vi "_Remote Communicate.vi"(4 "String":string, 5 "Max Mass":dbl, 6 "error in (no error)":errorcluster, 7 "DC Param":u16, 8 "Parameter":T1 {"Expt"."Mass Range"."Resolution Type" items=["High/High", "Medium/Medium", "Low/Low", "High/Medium", "High/Low", "Medium/High", "Medium/Low", "Low/High", "Low/Medium"]}, 9 "Command":T7=enum."Get Info") -> (0 "error out":errorcluster, 1 "Data Array":i32[](array[numeric]), 2 "Info":string, 3 "CommErr":bool)   [LabVIEW 2015]
uses:
  Type/_RT Data.ctl
  Type/_RT Command.ctl
  Type/_RT Parameter.ctl
  Type/_RT Active Ch.ctl
  Type/_RT Expt.ctl
  Type/_Run Mode.ctl
  Type/_RT Mass Range.ctl
  Type/_RT Res Type.ctl
  Type/TCP Packet Info.ctl
  Type/_File Command.ctl
  Type/_RT Configuration 2.ctl
  Type/_Log Command.ctl
  Configuration/_Global Configuration.vi
  <vilib>/Utility/config.llb/Read Key (String).vi
  <vilib>/Utility/config.llb/NI_LVConfig.lvlib
panel:
  out "Boolean":bool
  in  "Data":T8
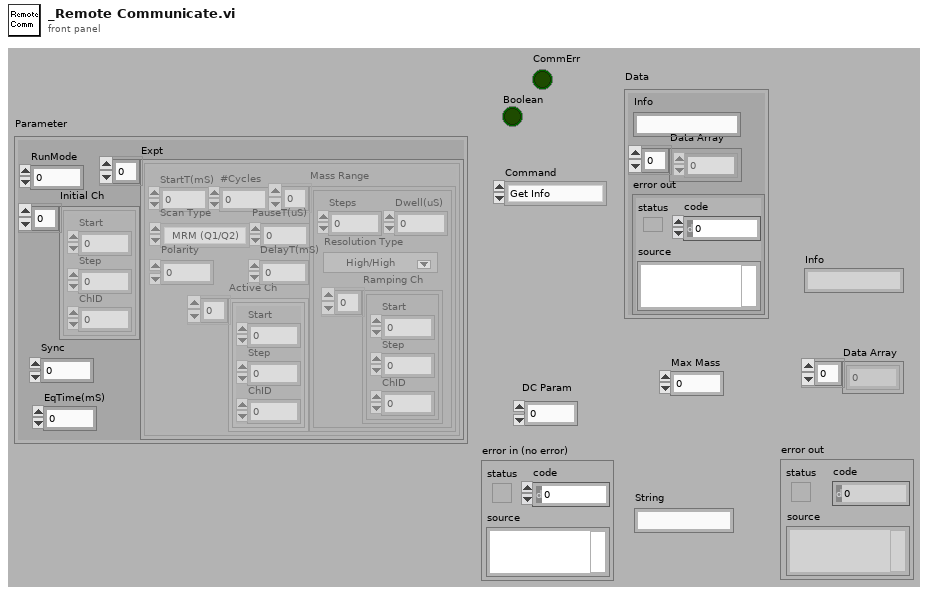
[diagram p1: front panel]
types:
  T1 = typedef "_RT Parameter.ctl" = cluster{"RunMode":i32, "Initial Ch":T2[], "Sync":u8, "Expt":T3[], "EqTime(mS)":i32}
  T2 = typedef "_RT Active Ch.ctl" = cluster{"Start":i32, "Step":i32, "ChID":i32}
  T3 = typedef "_RT Expt.ctl" = cluster{"StartT(mS)":i32, "#Cycles":i32, "Scan Type":T4, "PauseT(uS)":i32, "Polarity":u8, "DelayT(mS)":i32, "Active Ch":T2[], "Mass Range":T5[]}
  T4 = typedef "_Run Mode.ctl" = enum16{"MRM (Q1/Q2)", "Q1 Scan", "Q1 SRM", "Q2 Scan", "Q2 SRM", "Product Scan", "Precursor Scan", "Neutral Loss", "Neutral Gain"}
  T5 = typedef "_RT Mass Range.ctl" = cluster{"Steps":i32, "Dwell(uS)":i32, "Resolution Type":T6, "Ramping Ch":T2[]}
  T6 = typedef "_RT Res Type.ctl" = u16
  T7 = typedef "_RT Command.ctl" = enum16{"xml Start Run", "xml Start Actual Run", "xml Stop Run", "xml Runtime Update", "xml Get Status", "xml Get Table", "xml Set Table", "xml Get Configuration", "xml System Status", "xml Set LC Input Logic", "xml Get Data", "xml Get Info", "Start", "StartActualRun", "Stop", "Runtime Update", "Get Data", "Get Info", "Get Status", "Get Param", "Get Config", "Get Table", "Read ADC", "Set Oscillator", "Update Config", "Update Table", "Set All Pol", "Set Pol and DC", "Set Max Mass", "Toggle RP", "Toggle EL", "Set PIC", "Initialize Turbo", "Send Turbo Comm", "Close Turbo", "P1", "P2", "P3", "Send Serial", "Set LC Out", "Get LC In", "Read VAC", "Test Table", "Toggle Power", "Get Startup", "Set Startup", "Get ADC Table", "Set ADC Table", "Get Brief Status", "Get Detail Status", "Auxiliary Update", "Set CC Logics", "Set CC Input Logics", "Ignore Error", "invalid"}
  T8 = typedef "_RT Data.ctl" = cluster{"Info":string, "Data Array":i32[], "error out":errorcluster}
  T9 = typedef "TCP Packet Info.ctl" = cluster{"Packet Signature":string, "Sequence Number":i32, "Command":T7, "Data Message Size":u32, "Data Message Size":string, "Data Message":string, "Error Message Size":u32, "Error Message Size":string, "Error Message":string, "Checksum":u32, "Error Message":errorcluster, "Command ID":string}
  T10 = typedef "_File Command.ctl" = enum16{"No Command", "Open", "Open Read", "Write", "Get Spectrum", "Close"}
  T11 = typedef "_RT Configuration 2.ctl" = cluster{"Name":string, "Ch#":u8, "Min":dbl, "Max":dbl, "Def+":dbl, "Def-":dbl, "Offset":dbl, "Slope":dbl, "Type":u8, "Description":string, "SettleT":dbl}
  T12 = typedef "_RT Instrument 2.ctl" = cluster{"Table":T11[], "Instrument":string[]}
  T13 = typedef "NI_LVConfig.lvlib/Config Data RefNum.ctl" = refnum<k1>
  T14 = typedef "_Log Command.ctl" = enum16{"No Command", "Open", "Read", "Write", "Close", "Check Size"}
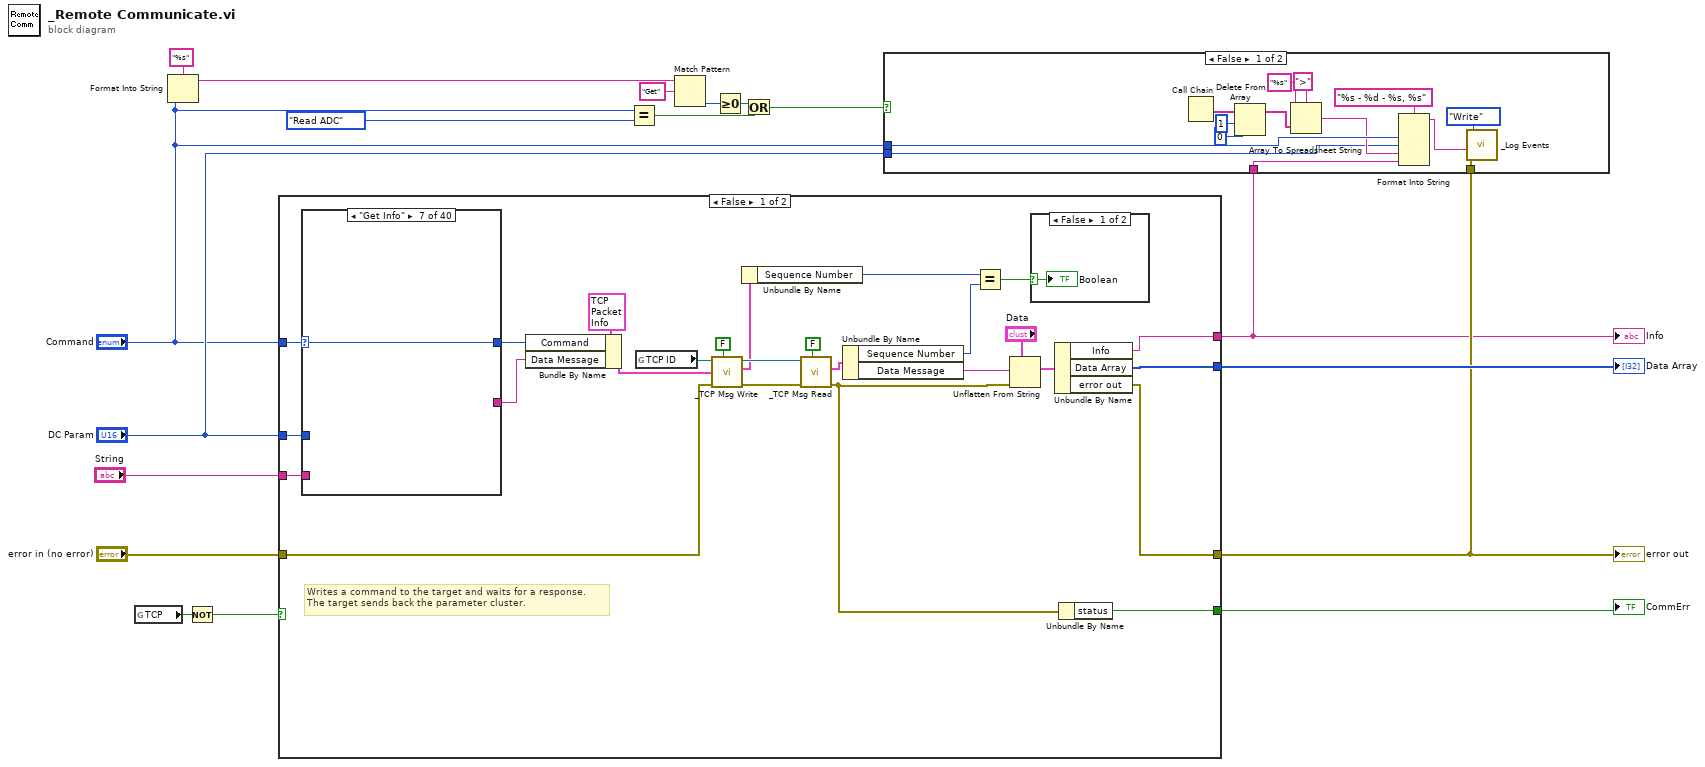
[diagram p0: block diagram]
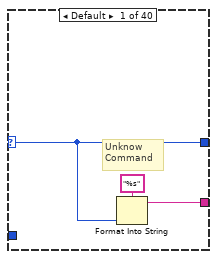
[diagram p4: hidden frame]
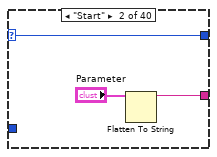
[diagram p5: hidden frame]
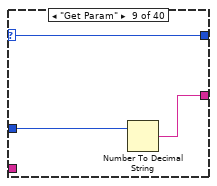
[diagram p11: hidden frame]
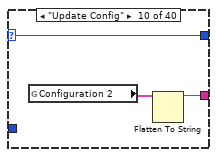
[diagram p12: hidden frame]
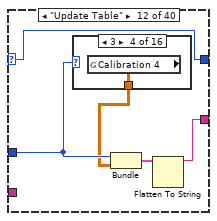
[diagram p14: hidden frame]
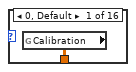
[diagram p15: hidden frame]
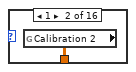
[diagram p16: hidden frame]
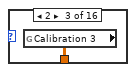
[diagram p17: hidden frame]
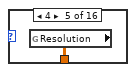
[diagram p18: hidden frame]
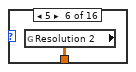
[diagram p19: hidden frame]
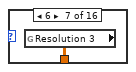
[diagram p20: hidden frame]
diagram:
  n1 = global read "_Global Configuration.vi" "TCP"() -> (w18:bool)
  n2 = Format Into String(format string="%s", "Command") -> (resulting string=w10:string)  [unwired: 2 in, 1 out]
  n3 = Not(x=w18) -> (.not. x?=w15:bool)
  n4 = case shown="False" w15 {
    selector: w15 -> [_ w151]
    tunnel: [w37 w156] -> w14
    tunnel: "error in (no error)" -> [w33 w156]
    tunnel: [w40 w154] -> w12
    tunnel: [w39 w153] -> w16
    tunnel: "Command" -> [w31 w155]
    tunnel: "DC Param" -> [w38 w152]
    tunnel: [w36 w151] -> w2
    tunnel: "String" -> [w35 _]
    frame False {
      # "Writes a command to the target and waits for a response.\nThe target sends back the parameter cluster."
      n5 = case shown="\"Get Info\"" w31 {
        selector: w31 -> [w46 w49 w52 w53 w54 w56 w57 w58 w59 w62 w65 w66 w87 w90 w92 w93 w94 w96 w98 w99 w102 w105 w108 w111 w114 w115 w118 w121 w124 w126 w128 w131 w134 w137 w138 w140 w141 w143 w145 w148]
        tunnel: [w47 w51 _ _ w55 _ _ _ w60 w63 _ w70 w88 w91 _ _ w95 w97 _ w100 w103 w107 w110 w113 _ w116 w119 w122 w125 w127 w130 w133 w136 _ w139 _ w142 w144 w147 w149] -> w29
        tunnel: w38 -> [_ _ _ _ _ _ _ _ w61 _ _ w68 w89 _ _ _ _ _ _ w101 w104 w106 w109 w112 _ w117 w120 w123 _ _ w129 w132 w135 _ _ _ _ _ _ w150]
        tunnel: w35 -> [_ _ _ _ w55 _ _ _ _ _ _ _ _ w91 _ _ w95 w97 _ _ _ _ _ _ _ _ _ _ w125 w127 _ _ _ _ w139 _ w142 w144 _ _]
        tunnel: [w46 w49 w52 w53 w54 w56 w57 w58 w59 w62 w65 w66 w87 w90 w92 w93 w94 w96 w98 w99 w102 w105 w108 w111 w114 w115 w118 w121 w124 w126 w128 w131 w134 w137 w138 w140 w141 w143 w145 w148] -> w28
        frame Default {
          # "Unknow\nCommand"
          n6 = Format Into String(format string="%s", w46) -> (resulting string=w47:string)  [unwired: 2 in, 1 out]
        }
        frame "Start" {
          n7 = Flatten To String(anything="Parameter") -> (data string=w51:string)  [unwired: 1 in, 4 out]
        }
        frame "StartActualRun" {
        }
        frame "Stop" {
        }
        frame "Runtime Update" {
        }
        frame "Get Data" {
        }
        frame "Get Info" {
        }
        frame "Get Status" {
        }
        frame "Get Param" {
          n8 = Number To Decimal String(number=w61) -> (decimal integer string=w60:string)  [unwired: 1 out]
        }
        frame "Update Config" {
          n9 = global read "_Global Configuration.vi" "Configuration 2"() -> (w64:T12)
          n10 = Flatten To String(anything=w64) -> (data string=w63:string)  [unwired: 1 in, 4 out]
        }
        frame "Get Config" {
        }
        frame "Update Table" {
          n11 = case shown="3" w68 {
            tunnel: [w71 w72 w73 w74 w75 w76 w77 w78 w79 w80 w81 w82 w83 w84 w85 w86] -> w67
            frame 0, Default {
              n12 = global read "_Global Configuration.vi" "Calibration"() -> (w71:dbl[][])
            }
            frame 1 {
              n13 = global read "_Global Configuration.vi" "Calibration 2"() -> (w72:dbl[][])
            }
            frame 2 {
              n14 = global read "_Global Configuration.vi" "Calibration 3"() -> (w73:dbl[][])
            }
            frame 3 {
              n15 = global read "_Global Configuration.vi" "Calibration 4"() -> (w74:dbl[][])
            }
            frame 4 {
              n16 = global read "_Global Configuration.vi" "Resolution"() -> (w75:dbl[][])
            }
            frame 5 {
              n17 = global read "_Global Configuration.vi" "Resolution 2"() -> (w76:dbl[][])
            }
            frame 6 {
              n18 = global read "_Global Configuration.vi" "Resolution 3"() -> (w77:dbl[][])
            }
            frame 7 {
              n19 = global read "_Global Configuration.vi" "Resolution 4"() -> (w78:dbl[][])
            }
            frame 8 {
              n20 = global read "_Global Configuration.vi" "Resolution 5"() -> (w79:dbl[][])
            }
            frame 9 {
              n21 = global read "_Global Configuration.vi" "Resolution 6"() -> (w80:dbl[][])
            }
            frame 10 {
              n22 = global read "_Global Configuration.vi" "Resolution 7"() -> (w81:dbl[][])
            }
            frame 11 {
              n23 = global read "_Global Configuration.vi" "Resolution 8"() -> (w82:dbl[][])
            }
            frame 12 {
              n24 = global read "_Global Configuration.vi" "Resolution 9"() -> (w83:dbl[][])
            }
            frame 13 {
              n25 = global read "_Global Configuration.vi" "Resolution 10"() -> (w84:dbl[][])
            }
            frame 14 {
              n26 = global read "_Global Configuration.vi" "Resolution 11"() -> (w85:dbl[][])
            }
            frame 15 {
              n27 = global read "_Global Configuration.vi" "Resolution 12"() -> (w86:dbl[][])
            }
          }
          n28 = Bundle("DC Param"=w68, "Resolution 12"=w67) -> (w69:cluster{"DC Param":u16, "Resolution 12":dbl[][]})  [unwired: 1 out]
          n29 = Flatten To String(anything=w69) -> (data string=w70:string)  [unwired: 1 in, 4 out]
        }
        frame "Get Table" {
          n30 = Number To Decimal String(number=w89) -> (decimal integer string=w88:string)  [unwired: 1 out]
        }
        frame "Set ADC Table" {
        }
        frame "Get ADC Table" {
        }
        frame "Read ADC" {
        }
        frame "Set Oscillator" {
        }
        frame "Set Startup" {
        }
        frame "Get Startup" {
        }
        frame "Set All Pol" {
          n31 = Type Cast(x=w101) -> (*(type *) &x=w100:string)  [unwired: 1 out]
        }
        frame "Set Pol and DC" {
          n32 = Type Cast(x=w104) -> (*(type *) &x=w103:string)  [unwired: 1 out]
        }
        frame "P1" {
          n33 = Type Cast(x=w106) -> (*(type *) &x=w107:string)  [unwired: 1 out]
        }
        frame "P2" {
          n34 = Type Cast(x=w109) -> (*(type *) &x=w110:string)  [unwired: 1 out]
        }
        frame "P3" {
          n35 = Type Cast(x=w112) -> (*(type *) &x=w113:string)  [unwired: 1 out]
        }
        frame "Read VAC" {
        }
        frame "Toggle Power" {
          n36 = Number To Decimal String(number=w117) -> (decimal integer string=w116:string)  [unwired: 1 out]
        }
        frame "Toggle RP" {
          n37 = Number To Decimal String(number=w120) -> (decimal integer string=w119:string)  [unwired: 1 out]
        }
        frame "Toggle EL" {
          n38 = Number To Decimal String(number=w123) -> (decimal integer string=w122:string)  [unwired: 1 out]
        }
        frame "Set PIC" {
        }
        frame "Send Serial" {
        }
        frame "Set LC Out" {
          n39 = Type Cast(x=w129) -> (*(type *) &x=w130:string)  [unwired: 1 out]
        }
        frame "Set CC Logics" {
          n40 = Type Cast(x=w132) -> (*(type *) &x=w133:string)  [unwired: 1 out]
        }
        frame "Set CC Input Logics" {
          n41 = Type Cast(x=w135) -> (*(type *) &x=w136:string)  [unwired: 1 out]
        }
        frame "Get LC In" {
        }
        frame "Get Brief Status" {
        }
        frame "Get Detail Status" {
        }
        frame "Auxiliary Update" {
        }
        frame "Test Table" {
        }
        frame "Set Max Mass" {
          n42 = Type Cast(x="Max Mass") -> (*(type *) &x=w147:string)  [unwired: 1 out]
        }
        frame "Ignore Error" {
          n43 = Number To Decimal String(number=w150) -> (decimal integer string=w149:string)  [unwired: 1 out]
        }
      }
      n44 = Bundle By Name(cluster=T9 {"Packet Signature"="", "Sequence Number"=0, "Command"=enum."xml Set LC Input Logic", "Data Message Size"=0, "Data Message Size"="", "Data Message"="", "Error Message Size"=0, "Error Message Size"="", "Error Message"="", "Checksum"=0, "Error Message"={"status"=FALSE, "code"=0, "source"=""}, "Command ID"=""} ("Packet Info In"), "Command"=w28, "Data Message"=w29) -> (w27:T9)
      n45 = global read "_Global Configuration.vi" "TCP ID"() -> (w44:refnum<k5>)
      n46 = call "_TCP Msg Write.vi"("RT"=FALSE, "error in"=w33, "Packet Info In"=w27, "connection ID In"=w44) -> ("error out"=w21:errorcluster, "Packet Info In Out"=w22:T9, "connection ID out"=w42:refnum<k5>)  [unwired: 1 in, 4 out]
      n47 = Unbundle By Name(w22) -> ("Sequence Number"=w25:i32)
      n48 = call "_TCP Msg Read.vi"("RT"=FALSE, "error in"=w21, "connection ID"=w42) -> ("error out"=w19:errorcluster, "Packet Info"=w20:T9)  [unwired: 2 in, 5 out]
      n49 = Unbundle By Name(w20) -> ("Sequence Number"=w24:i32, "Data Message"=w34:string)
      n50 = Equal?(x=w25, y=w24) -> (x = y?=w23:bool)
      n51 = Unflatten From String(type="Data", binary string=w34, error in (no error)=w19) -> (value=w41:T8)  [unwired: 4 out]
      n52 = case shown="False" w23 {
        selector: w23 -> [w45 _]
        frame False {
          "Boolean" <- w45
        }
        frame True {
        }
      }
      n53 = Unbundle By Name(w41) -> ("Info"=w40:string, "Data Array"=w39:i32[], "error out"=w37:errorcluster)
      n54 = Unbundle By Name(w19) -> ("status"=w36:bool)
    }
    frame True {
      # "For simulation"
      n55 = case shown="\"Get Status\"" w155 {
        tunnel: [_ _ "Ionica is running in simulation mode.\n(System is idling: 00h00m00s)" w164 w172 "0\t118061205\tSimilated FPGA is idling\r\n4\t0\tFIFO Mis-Read #\r\n5\t4228\t# of Recorded Data Points\r\n6\t1451\tTime to Prepare Next Cycle (ticks)\r\n7\t14\tTotal # of Experiments Ran\r\n0\t1\tSingle Mode\r\n1\t10\t# of Active Channels\r\n2\t1000000\tHigh Level Time (uS)\r\n3\t500000\tLow Level Time (uS)" ("Info") w190 _ w199 w209] -> w154
        tunnel: [_ w157 _ _ _ _ _ w192 _ _] -> w153
        tunnel: w152 -> [_ _ _ _ w171 _ _ _ _ _]
        frame Default {
        }
        frame "Get Data" {
          n56 = call "_File Server Simulation.vi"("FileCommand"=_File_Command."Get Spectrum") -> ("DataArray"=w157:i32[])  [unwired: 1 in, 1 out]
        }
        frame "Get Info" {
        }
        frame "Get Status" {
          n57 = global read "_Global Configuration.vi" "Run"() -> (w168:bool)
          n58 = global read "_Global Configuration.vi" "Acquiring"() -> (w160:bool)
          n59 = Select(t="1: Simulated FPGA is running" ("regular expression"), s=w168, f="0: Simulated FPGA is in idle state" ("regular expression")) -> (s? t:f=w165:string)
          n60 = Select(t="Running" ("regular expression"), s=w160, f="Ready" ("regular expression")) -> (s? t:f=w161:string)
          n61 = Format Into String(format string="%s.  Instr State = %s.", w165, w161) -> (resulting string=w164:string)  [unwired: 2 in, 1 out]
        }
        frame "Get Table" {
          n62 = case shown="6" w171 {
            tunnel: [w173 w174 w175 w176 w177 w178 w179 w180 w181 w182 w183 w184 w185 w186 w187 w188] -> w170
            frame 0, Default {
              n63 = global read "_Global Configuration.vi" "Calibration"() -> (w173:dbl[][])
            }
            frame 1 {
              n64 = global read "_Global Configuration.vi" "Calibration 2"() -> (w174:dbl[][])
            }
            frame 2 {
              n65 = global read "_Global Configuration.vi" "Calibration 3"() -> (w175:dbl[][])
            }
            frame 3 {
              n66 = global read "_Global Configuration.vi" "Calibration 4"() -> (w176:dbl[][])
            }
            frame 4 {
              n67 = global read "_Global Configuration.vi" "Resolution"() -> (w177:dbl[][])
            }
            frame 5 {
              n68 = global read "_Global Configuration.vi" "Resolution 2"() -> (w178:dbl[][])
            }
            frame 6 {
              n69 = global read "_Global Configuration.vi" "Resolution 3"() -> (w179:dbl[][])
            }
            frame 7 {
              n70 = global read "_Global Configuration.vi" "Resolution 4"() -> (w180:dbl[][])
            }
            frame 8 {
              n71 = global read "_Global Configuration.vi" "Resolution 5"() -> (w181:dbl[][])
            }
            frame 9 {
              n72 = global read "_Global Configuration.vi" "Resolution 6"() -> (w182:dbl[][])
            }
            frame 10 {
              n73 = global read "_Global Configuration.vi" "Resolution 7"() -> (w183:dbl[][])
            }
            frame 11 {
              n74 = global read "_Global Configuration.vi" "Resolution 8"() -> (w184:dbl[][])
            }
            frame 12 {
              n75 = global read "_Global Configuration.vi" "Resolution 9"() -> (w185:dbl[][])
            }
            frame 13 {
              n76 = global read "_Global Configuration.vi" "Resolution 10"() -> (w186:dbl[][])
            }
            frame 14 {
              n77 = global read "_Global Configuration.vi" "Resolution 11"() -> (w187:dbl[][])
            }
            frame 15 {
              n78 = global read "_Global Configuration.vi" "Resolution 12"() -> (w188:dbl[][])
            }
          }
          n79 = Flatten To String(anything=w170) -> (data string=w172:string)  [unwired: 1 in, 4 out]
        }
        frame "Get Param" {
        }
        frame "Get Config" {
          n80 = global read "_Global Configuration.vi" "Configuration 2"() -> (w191:T12)
          n81 = Flatten To String(anything=w191) -> (data string=w190:string)  [unwired: 1 in, 4 out]
        }
        frame "Read ADC" {
          n82 = for {
            N: 128 -> [_]
            tunnel: [w194] -> w192 mode=indexing
            n83 = Random Number (0-1)() -> (number: 0 to 1=w197:dbl)
            n84 = Multiply(x=w197, y=4096.0) -> (x*y=w195:dbl)
            n85 = To Long Integer(number=w195) -> (32bit integer=w194:i32)
          }
        }
        frame "Get Detail Status" {
          n86 = global read "_Global Configuration.vi" "Single Source"() -> (w201:bool)
          n87 = Select(t="<Data>\n<SystemStatus>\nInstrument State=Simulation;\nServer State=0;\nLC1 IN=0;\nLC2 IN=0;\nLC1 Out1=1;\nLC1 Out2=0;\nLC2 Out1=1;\nLC2 Out2=0;\nSystem Error=;\nVacuum Gauge=1;\nVacuum Pressure=1164.34;\nVacuum Error=No Error;\nForeline Pressure=-29.22;\nForeline Error=No Error;\nSource 1=ESI;\nNeb Gas1=385.03;\nAux Gas1=313.04;\nCurtain Gas=109.38;\nCC Gas=439.94;\nOut of Gas=0;\nHSID Temp=198.00;\nSource1 Temp=251.00;\nVoltage Output=1;\nExhaust Pressure=3752.31;\nQ2RF HS1 Temp=36.38;\nQ1RF HS1 Temp=40.53;\nM1RF HS1 Temp=37.11;\nQ2RF HS2 Temp=37.35;\nQ1RF HS2 Temp=40.77;\nM1RF HS2 Temp=36.62;\nCorona Current=0.00;\nHTR PS Current=8.23;\nQ1 Tuning DC=-7.15;\nQ2 Tuning DC=-8.26;\nM1RF Tuning DC=-5.58;\nDoor Interlock=1;\n24V=24;\n28V=28;\n-28V=-28;\n60V=59;\n15V=15;\n-15V=-15;\nLens Board 2 +5V=5;\nLens Board 2 -5V=-5;\nLens Board 1 +5V=5;\nLens Board 1 -5V=-5;\nSource Exhaust Valve=1;\n</SystemStatus>\n<Log>\n97:33:2, Starting Up\n97:33:3, Electronics ON\n97:33:11, System Pumping Down\n97:34:28, Roughing Pump Standby\n97:34:28, Turbo Startup\n97:34:31, Turbo Ready\n97:34:34, System Ready\n</Log>\n</Data>", s=w201, f="<Data>\n<SystemStatus>\nInstrument State=Simulation;\nServer State=0;\nLC1 IN=0;\nLC2 IN=0;\nLC1 Out1=1;\nLC1 Out2=0;\nLC2 Out1=1;\nLC2 Out2=0;\nSystem Error=;\nVacuum Gauge=1;\nVacuum Pressure=1164.34;\nVacuum Error=No Error;\nForeline Pressure=-29.22;\nForeline Error=No Error;\nSource 1=ESI;\nSource 2=APCI;\nNeb Gas1=385.03;\nNeb Gas2=0.00;\nAux Gas1=313.04;\nAux Gas2=0.00;\nCurtain Gas=109.38;\nCC Gas=439.94;\nOut of Gas=0;\nHSID Temp=198.00;\nSource1 Temp=251.00;\nSource2 Temp=106.00;\nVoltage Output=1;\nExhaust Pressure=3752.31;\nQ2RF HS1 Temp=36.38;\nQ1RF HS1 Temp=40.53;\nM1RF HS1 Temp=37.11;\nQ2RF HS2 Temp=37.35;\nQ1RF HS2 Temp=40.77;\nM1RF HS2 Temp=36.62;\nCorona Current=0.00;\nHTR PS Current=8.23;\nQ1 Tuning DC=-7.15;\nQ2 Tuning DC=-8.26;\nM1RF Tuning DC=-5.58;\nDoor Interlock=1;\n24V=24;\n28V=28;\n-28V=-28;\n60V=59;\n15V=15;\n-15V=-15;\nLens Board 2 +5V=5;\nLens Board 2 -5V=-5;\nLens Board 1 +5V=5;\nLens Board 1 -5V=-5;\nSource Exhaust Valve=1;\n</SystemStatus>\n<Log>\n97:33:2, Starting Up\n97:33:3, Electronics ON\n97:33:11, System Pumping Down\n97:34:28, Roughing Pump Standby\n97:34:28, Turbo Startup\n97:34:31, Turbo Ready\n97:34:34, System Ready\n</Log>\n</Data>") -> (s? t:f=w199:string)
        }
        frame "Get ADC Table" {
          n88 = call "_Open Preference File.vi"() -> ("error"=w205:errorcluster, "refnum"=w204:T13)  [unwired: 3 in, 3 out]
          n89 = for {
            N: 128 -> [_]
            tunnel: w204 -> [w218]
            tunnel: w205 -> [w217]
            tunnel: "ADC" ("section") -> [w216]
            tunnel: [w214] -> w208
            tunnel: [w212] -> w202 mode=indexing
            i -> [w213]
            n90 = for {
              N: 8 -> [_]
              tunnel: w218 -> [w228]
              tunnel: w217 -> [w227]
              tunnel: w216 -> [w220]
              tunnel: [w226] -> w214
              tunnel: w213 -> [w224]
              tunnel: [w221] -> w212 mode=indexing
              i -> [w225]
              n91 = Format Into String(format string="Row%d-Col%d" ("section"), w224, w225) -> (resulting string=w222:string)  [unwired: 2 in, 1 out]
              n92 = call-poly <vilib>:"Read Key.vi"("section"=w220, "error in (no error)"=w227, "default value"="", "key"=w222, "refnum"=w228) -> ("value"=w221:string, "refnum out"=w226:T13)  [unwired: 3 in, 2 out]
            }
          }
          n93 = call <vilib>:"Close Config Data.vi"("write file if changed (T)"=FALSE ("write configuration file? (T)"), "refnum"=w208) -> ()  [unwired: 8 in, 2 out]
          n94 = for {
            tunnel: w202 -> [w240] mode=indexing
            tunnel: T11 {"Name"="", "Ch#"=0, "Min"=0.0, "Max"=0.0, "Def+"=0.0, "Def-"=0.0, "Offset"=0.0, "Slope"=0.0, "Type"=0, "Description"="", "SettleT"=0.0} ("Configuration") -> [w235]
            tunnel: [w229] -> w211 mode=indexing
            n95 = Index Array(array=w240) -> (element #2=w234:string, element #4=w239:string, element #5=w238:string, element #7=w237:string, element #8=w236:string)  [unwired: 8 in, 3 out]
            n96 = Fract/Exp String To Number(string=w239) -> (number=w233:dbl)  [unwired: 4 out]
            n97 = Fract/Exp String To Number(string=w238) -> (number=w232:dbl)  [unwired: 4 out]
            n98 = Fract/Exp String To Number(string=w237) -> (number=w231:dbl)  [unwired: 4 out]
            n99 = Fract/Exp String To Number(string=w236) -> (number=w230:dbl)  [unwired: 4 out]
            n100 = Bundle By Name(cluster=w235, "Name"=w234, "Offset"=w233, "Slope"=w232, "Min"=w231, "Max"=w230) -> (w229:T11)
          }
          n101 = Flatten To String(anything=w211) -> (data string=w209:string)  [unwired: 1 in, 4 out]
        }
      }
    }
  }
  "error out" <- w14
  "Data Array" <- w16
  "Info" <- w12
  "CommErr" <- w2
  n102 = Equal?(x="Command", y=_RT_Command."Read ADC") -> (x = y?=w4:bool)
  n103 = Match Pattern(string=w10, regular expression="Get") -> (offset past match=w8:i32)  [unwired: 4 out]
  n104 = Greater Or Equal To 0?(x=w8) -> (x >= 0?=w5:bool)
  n105 = Or(x=w5, y=w4) -> (x .or. y?=w3:bool)
  n106 = case shown="False" w3 {
    tunnel: "Command" -> [w254 _]
    tunnel: w14 -> [w252 _]
    tunnel: "DC Param" -> [w242 _]
    tunnel: w12 -> [w241 _]
    frame False {
      n107 = Call Chain() -> (call chain=w247:string[])
      n108 = Delete From Array(array=w247, length=1, index=0) -> (array with subset deleted=w244:string[])  [unwired: 1 out]
      n109 = Array To Spreadsheet String(delimiter (Tab)=">", array=w244, 3:"%s" ("format string")) -> (spreadsheet string=w243:string)
      n110 = Format Into String(format string="%s - %d - %s, %s", w254, w242, w243, w241) -> (resulting string=w251:string)  [unwired: 2 in, 1 out]
      n111 = call "_Log Events.vi"("error in (no error)"=w252, "Event"=w251, "Log Command"=_Log_Command."Write" ("File Command")) -> ()  [unwired: 5 in, 2 out]
    }
    frame True {
    }
  }
